vi "Log_SetUserComment.vi"() -> ()   [LabVIEW 2012]
uses:
  GlobalVariables_DIALMain.vi
panel:
  in  "Cancel":bool
  in  "User":string="Robert"
  in  "Comment":string
  in  "Set Status":bool
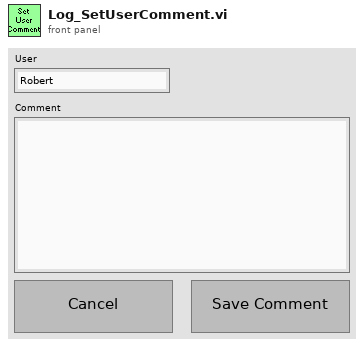
[diagram p1: front panel]
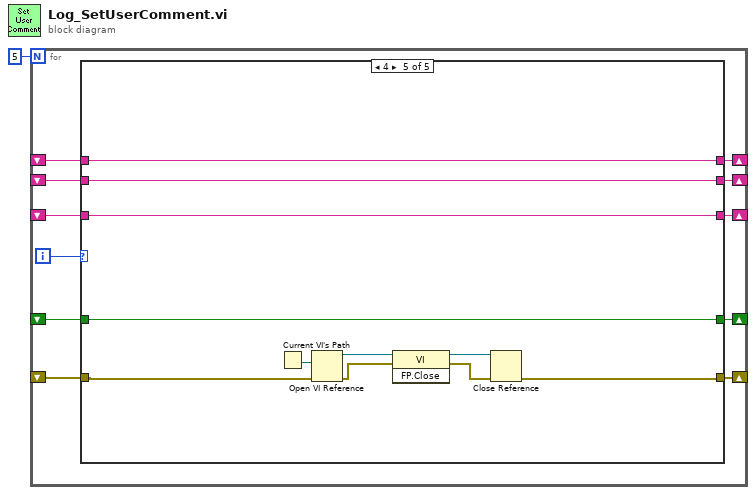
[diagram p0: block diagram]
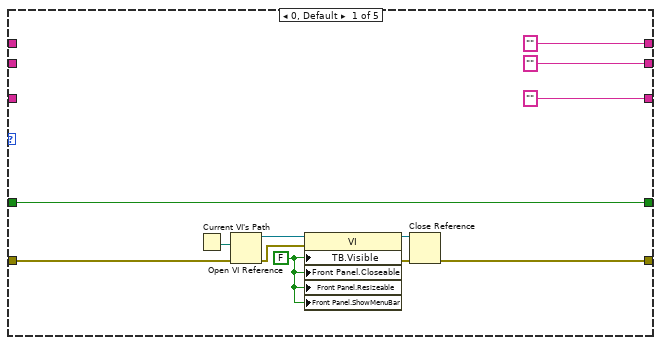
[diagram p2: hidden frame]
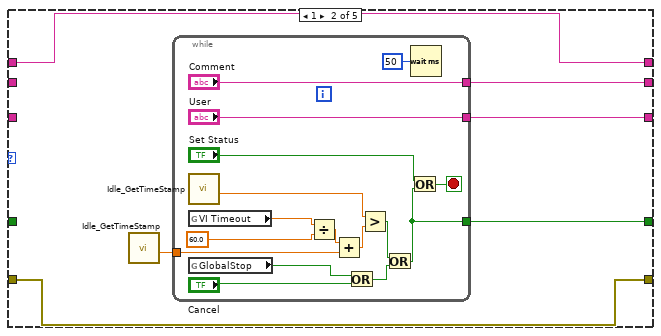
[diagram p3: hidden frame]
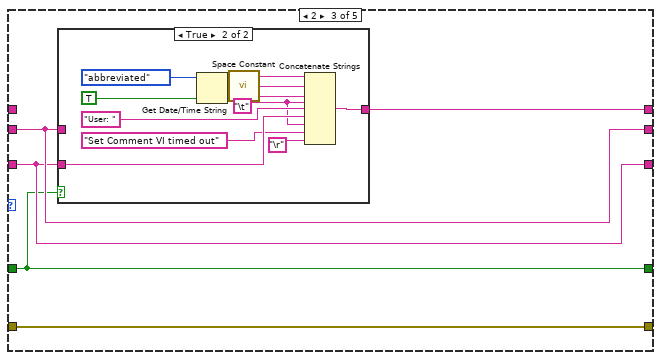
[diagram p4: hidden frame]
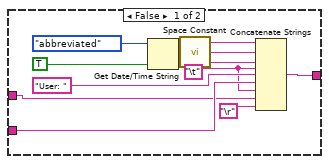
[diagram p5: hidden frame]
diagram:
  n1 = for {
    N: 5 -> [_]
    shift-right: [w11] -> _
    shift-left: _ -> [w7]
    shift-right: [w10] -> _
    shift-left: _ -> [w6]
    shift-right: [w9] -> _
    shift-left: _ -> [w8]
    shift-right: [w5] -> _
    shift-left: _ -> [w4]
    shift-right: [w2] -> _
    shift-left: _ -> [w3]
    i -> [w12]
    n2 = case shown="4" w12 {
      tunnel: ["" ("Comment") w29 w51 w78 w88] -> w11
      tunnel: ["" ("User") w28 w50 w77 w87] -> w10
      tunnel: [w16 w27 w49 w76 w86] -> w9
      tunnel: w8 -> [w16 _ w49 w76 w86]
      tunnel: w7 -> [_ _ w51 w78 w88]
      tunnel: w6 -> [_ _ w50 w77 w87]
      tunnel: ["" w26 w48 w75 w89] -> w5
      tunnel: w4 -> [_ w26 _ w75 w89]
      tunnel: w3 -> [w14 w25 w47 w74 w80]
      tunnel: [w13 w25 w47 w74 w79] -> w2
      frame 0, Default {
        w24 = FALSE ("Tool Bar:Visible")
        n3 = Current VI's Path() -> (path=w19:path)
        n4 = Open VI Reference(vi path=w19, error in (no error)=w14) -> (vi reference=w20:refnum<vi>, error out=w21:errorcluster)  [unwired: 4 in]
        n5 = property class="VI"(reference=w20, error in=w21, "TB.Visible"=w24, "Front Panel.Closeable"=w24, "Front Panel.Resizeable"=w24, "Front Panel.ShowMenuBar"=w24) -> (reference out=w22:refnum<vi>, error out=w23:errorcluster)
        n6 = Close Reference(reference=w22, error in (no error)=w23) -> (error out=w13:errorcluster)
      }
      frame 1 {
        n7 = call "Idle_GetTimeStamp.vi"() -> ("Fractional Hours"=w30:dbl)  [unwired: 11 in]
        n8 = while {
          tunnel: ["Comment"] -> w29
          tunnel: ["User"] -> w28
          tunnel: w30 -> [w37]
          tunnel: [w35] -> w27
          stop <- w38 stop-if-true
          n9 = call "Idle_GetTimeStamp.vi"() -> ("Fractional Hours"=w43:dbl)  [unwired: 11 in]
          n10 = global read "GlobalVariables_DIALMain.vi" "VI Timeout"() -> (w32:dbl)
          n11 = global read "GlobalVariables_DIALMain.vi" "GlobalStop"() -> (w31:bool)
          n12 = Divide(x=w32, y=60.0) -> (x/y=w40:dbl)
          n13 = Add(x=w40, y=w37) -> (x+y=w42:dbl)
          n14 = Or(x=w31, y="Cancel") -> (x .or. y?=w33:bool)
          n15 = Greater?(x=w43, y=w42) -> (0:w36:bool)
          n16 = Or(x=w36, y=w33) -> (x .or. y?=w35:bool)
          n17 = Or(x="Set Status", y=w35) -> (x .or. y?=w38:bool)
          n18 = Wait (ms)(milliseconds to wait=u32 50) -> ()  [unwired: 1 out]
        }
      }
      frame 2 {
        n19 = case shown="True" w49 {
          tunnel: w51 -> [w54 _]
          tunnel: w50 -> [w55 w66]
          tunnel: [w57 w68] -> w48
          frame False {
            w53 = "\t"
            n20 = Get Date/Time String(date format (0)=enum16{"short", "long", "abbreviated"}."abbreviated", want seconds? (F)=TRUE) -> (date string=w61:string, time string=w60:string)  [unwired: 1 in]
            n21 = call <vilib>:"Space Constant.vi"() -> ("String"=w62:string)
            n22 = Concatenate Strings(w61, w62, w60, w53, "User: ", w55, w53, w54, "\r") -> (w57:string)
          }
          frame True {
            w65 = "\t"
            n23 = Get Date/Time String(date format (0)=enum16{"short", "long", "abbreviated"}."abbreviated", want seconds? (F)=TRUE) -> (date string=w72:string, time string=w71:string)  [unwired: 1 in]
            n24 = call <vilib>:"Space Constant.vi"() -> ("String"=w73:string)
            n25 = Concatenate Strings(w72, w73, w71, w65, "User: ", w66, w65, "Set Comment VI timed out" ("string"), "\r") -> (w68:string)
          }
        }
      }
      frame 3 {
      }
      frame 4 {
        n26 = Current VI's Path() -> (path=w85:path)
        n27 = Open VI Reference(vi path=w85, error in (no error)=w80) -> (vi reference=w84:refnum<vi>, error out=w83:errorcluster)  [unwired: 4 in]
        n28 = invoke on="Invoke Node" class="VI" method="FP.Close"(reference=w84, error in=w83) -> (reference out=w81:refnum<vi>, error out=w82:errorcluster)  [unwired: 1 in, 1 out]
        n29 = Close Reference(reference=w81, error in (no error)=w82) -> (error out=w79:errorcluster)
      }
    }
  }
